vi "test 4- normalModeCallsChainMode.vi"(8 "error in (no error)":errorcluster, 11 "TestCase in":refnum<class "testcase-SyncMessage.lvclass">) -> (0 "error out":errorcluster, 3 "TestCase out":refnum<class "testcase-SyncMessage.lvclass">)   [LabVIEW 2017, in "testcase-SyncMessage.lvclass"]
uses:
  testcase-SyncMessage.lvclass
  <vilib>/addons/_JKI Toolkits/VI Tester/TestCase.llb/TestCase.lvclass
  src/user.lib/_NEVSTOP/Communicable State Machine(CSM)/Communicable State Machine.lvlib
  C:/Program Files (x86)/National Instruments/LabVIEW 2017/vi.lib/addons/_JKI Toolkits/VI Tester/TestCase.llb/TestCase.lvclass
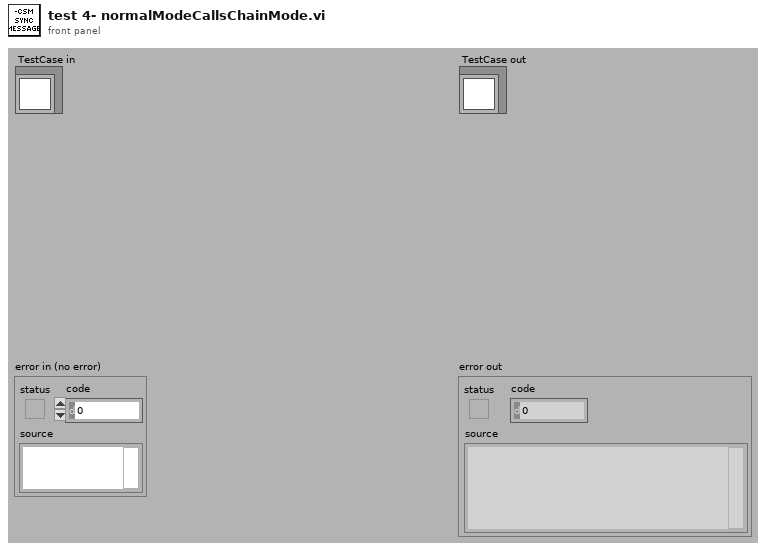
[diagram p1: front panel]
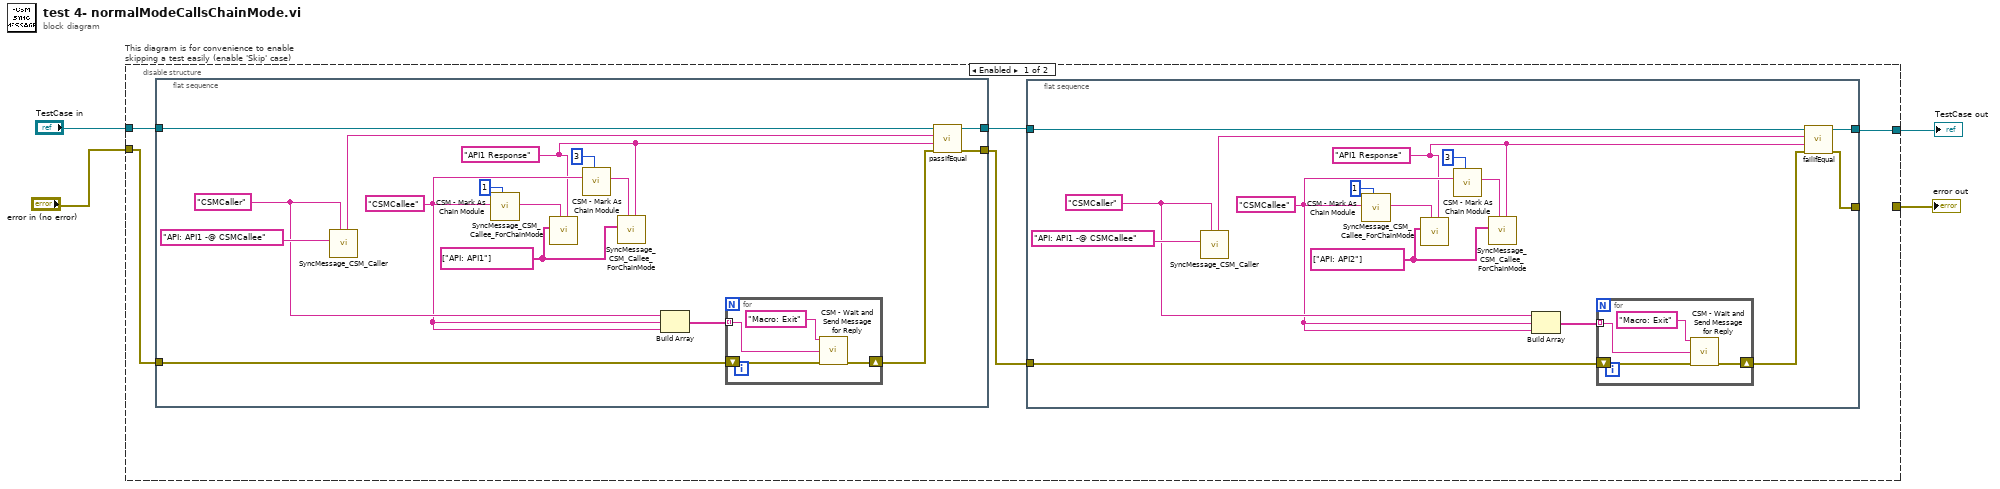
[diagram p0: block diagram]
diagram:
  n1 = disable-structure "This diagram is for convenience to enable skipping a test easily (enable 'Skip' case)" shown="Enabled" {
    disable-tunnel: "TestCase in" -> [w9 w53]
    disable-tunnel: [w6 w51] -> w2
    disable-tunnel: [_ w52] -> w1
    disable-tunnel: "error in (no error)" -> [w8 w50]
    frame Enabled {
      n2 = flat-sequence {
        tunnel: w9 -> [w45]
        tunnel: [w44] -> w7
        tunnel: [w43] -> w5
        tunnel: w8 -> [w30]
        frame #0 {
          w35 = string[] ["API: API1"] ("Allowed Messages (Empty for All)")
          w34 = "CSMCallee" ("CSMCallee")
          w39 = "CSMCaller" ("CSMCaller")
          w31 = "API1 Response" ("API response in")
          n3 = call "SyncMessage_CSM_Caller.vi"("Name (\"\" to Use UUID)"=w39, "Intermodule Message in"="API: API1 -@ CSMCallee") -> ("API received Response out"=w41:string)  [unwired: 9 in]
          n4 = call "CSM - Mark As Chain Module.vi"("Order"=1, "CSM Name"=w34) -> ("CSM Name (Marked As Chain)"=w36:string)  [unwired: 8 in]
          n5 = call "SyncMessage_CSM_Callee_ForChainMode.vi"("API response in"=w31, "Name (\"\" to Use UUID)"=w36, "Allowed Messages (Empty for All)"=w35) -> ()  [unwired: 9 in]
          n6 = call "CSM - Mark As Chain Module.vi"("Order"=3, "CSM Name"=w34) -> ("CSM Name (Marked As Chain)"=w32:string)  [unwired: 8 in]
          n7 = call "SyncMessage_CSM_Callee_ForChainMode.vi"("API response in"=w31, "Name (\"\" to Use UUID)"=w32, "Allowed Messages (Empty for All)"=w35) -> ()  [unwired: 9 in]
          n8 = Build Array(w39, w34, w34) -> (w40:string[])
          n9 = for {
            shift-right: [w47] -> w38
            shift-left: w30 -> [w48]
            tunnel: w40 -> [w46] mode=indexing
            n10 = call "CSM - Wait and Send Message for Reply.vi"("State"="Macro: Exit", "Target Module"=w46, "Error In (No Error)"=w48) -> ("error out"=w47:errorcluster)  [unwired: 10 in, 2 out]
          }
          n11 = call-dynamic "passIfEqual.vi"("error in (no error)"=w38, "y"=w31, "x"=w41, "TestCase in"=w45) -> ("error out"=w43:errorcluster, "TestCase out"=w44:refnum<class "testcase-SyncMessage.lvclass">)  [unwired: 6 in]
        }
      }
      n12 = flat-sequence {
        tunnel: w7 -> [w25]
        tunnel: [w24] -> w6
        tunnel: [w23] -> _
        tunnel: w5 -> [w10]
        frame #0 {
          w15 = string[] ["API: API2"] ("Allowed Messages (Empty for All)")
          w14 = "CSMCallee" ("CSMCallee")
          w19 = "CSMCaller" ("CSMCaller")
          w11 = "API1 Response" ("API response in")
          n13 = call "SyncMessage_CSM_Caller.vi"("Name (\"\" to Use UUID)"=w19, "Intermodule Message in"="API: API1 -@ CSMCallee") -> ("API received Response out"=w21:string)  [unwired: 9 in]
          n14 = call "CSM - Mark As Chain Module.vi"("Order"=1, "CSM Name"=w14) -> ("CSM Name (Marked As Chain)"=w16:string)  [unwired: 8 in]
          n15 = call "SyncMessage_CSM_Callee_ForChainMode.vi"("API response in"=w11, "Name (\"\" to Use UUID)"=w16, "Allowed Messages (Empty for All)"=w15) -> ()  [unwired: 9 in]
          n16 = call "CSM - Mark As Chain Module.vi"("Order"=3, "CSM Name"=w14) -> ("CSM Name (Marked As Chain)"=w12:string)  [unwired: 8 in]
          n17 = call "SyncMessage_CSM_Callee_ForChainMode.vi"("API response in"=w11, "Name (\"\" to Use UUID)"=w12, "Allowed Messages (Empty for All)"=w15) -> ()  [unwired: 9 in]
          n18 = Build Array(w19, w14, w14) -> (w20:string[])
          n19 = for {
            shift-right: [w27] -> w18
            shift-left: w10 -> [w28]
            tunnel: w20 -> [w26] mode=indexing
            n20 = call "CSM - Wait and Send Message for Reply.vi"("State"="Macro: Exit", "Target Module"=w26, "Error In (No Error)"=w28) -> ("error out"=w27:errorcluster)  [unwired: 10 in, 2 out]
          }
          n21 = call-dynamic "failIfEqual.vi"("error in (no error)"=w18, "y"=w11, "x"=w21, "TestCase in"=w25) -> ("error out"=w23:errorcluster, "TestCase out"=w24:refnum<class "testcase-SyncMessage.lvclass">)  [unwired: 6 in]
        }
      }
    }
    frame Disabled {
      # "skip test result while test is under development"
      n22 = call <vilib>:"skip.vi"("error in (no error)"=w50, "TestCase in"=w53) -> ("error out"=w52:errorcluster, "TestCase out"=w51:refnum<class "testcase-SyncMessage.lvclass">)  [unwired: 8 in]
    }
  }
  "error out" <- w1
  "TestCase out" <- w2
